vi "Set Magnet.vi"(4 "Mode":T2, 6 "Axis":T1, 8 "error in (no error)":errorcluster, 9 "Target Rate (T/min)":dbl, 10 "Target Field (T)":dbl, 11 "instrument.PPMS2 in":refnum<class "instrument.PPMS2.lvclass">) -> (0 "error out":errorcluster, 3 "instrument.PPMS2 out":refnum<class "instrument.PPMS2.lvclass">)   [LabVIEW 2019, in "instrument.PPMS2.lvclass"]
uses:
  instrument.PPMS2.lvclass
  <userlib>/LevyLab/Levylab Instruments/Instrument Types/Cryostat/Typedefs/Magnet Mode--Enum.ctl
  <userlib>/LevyLab/Levylab Instruments/Instrument Types/Cryostat/Typedefs/Magnet Axis--Enum.ctl
  Typedefs/PPMS2.Commands-enum.ctl
  <userlib>/LevyLab/Levylab Instruments/Instrument Types/Cryostat/Typedefs/Set Magnet--cluster.ctl
  d11e231a-c1e5-403b-8add-65da9e1ac210.vi
  d11e231a-c1e5-403b-8add-65da9e1ac210.vi/1872bd40-8905-4030-a4f5-2c54e5c49330.vi
  <userlib>/LevyLab/Levylab Instruments/SMOs/RemoteControl/API/Remote Client.vi
  <userlib>/LevyLab/Levylab Instruments/Instrument Types/Cryostat/Instrument.Cryostat.lvclass
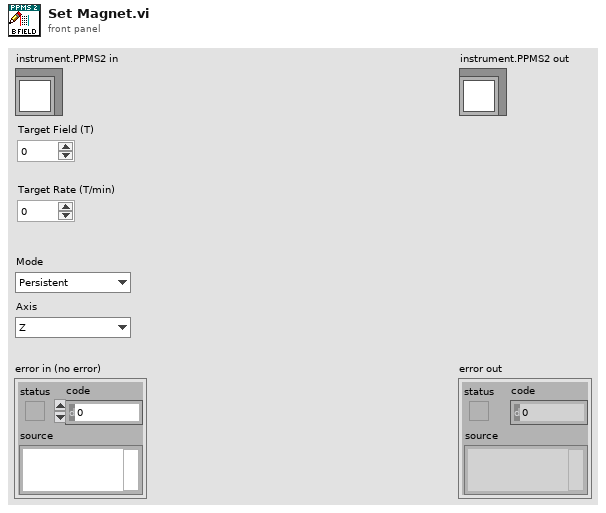
[diagram p1: front panel]
types:
  T1 = typedef "Instrument.Cryostat.lvclass/Magnet Axis--Enum.ctl" = enum16{"Z", "X", "Y"}
  T2 = typedef "Instrument.Cryostat.lvclass/Magnet Mode--Enum.ctl" = enum16{"Persistent", "Driven"}
  T3 = typedef "Instrument.Cryostat.lvclass/Set Magnet--cluster.ctl" = cluster{"Field (T)":dbl, "Rate (T/min)":dbl, "Axis":T1, "Mode":T2}
  T4 = typedef "instrument.PPMS2.lvclass/PPMS2.Commands-enum.ctl" = enum16{"Get Magnet Field", "Get Helium Level", "Get Temperature", "Get Angle", "Set Magnet Field", "Set Temperature", "Set Angle", "getAll"}
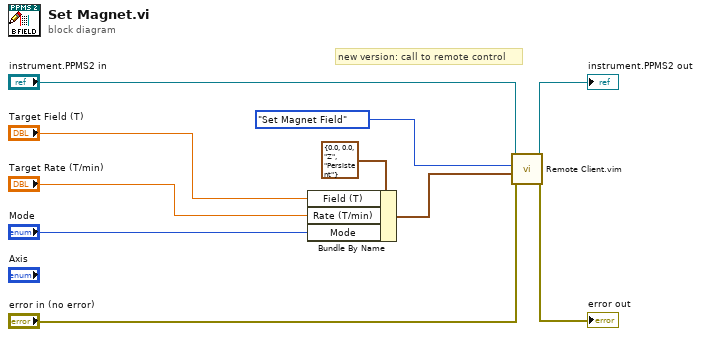
[diagram p0: block diagram]
diagram:
  # "new version: call to remote control"
  n1 = Bundle By Name(cluster=T3 {"Field (T)"=0.0, "Rate (T/min)"=0.0, "Axis"=enum."Z", "Mode"=enum."Persistent"} ("Set Magnet Field"), "Field (T)"="Target Field (T)", "Rate (T/min)"="Target Rate (T/min)", "Mode"="Mode") -> (w5:T3)
  n2 = call "Remote Client.vim"("error in (no error)"="error in (no error)", "Data"=w5, "Command"=PPMS2.Commands-enum."Set Magnet Field" ("Enum"), "Instrument in"="instrument.PPMS2 in") -> ("error out"=→"error out":errorcluster, "Instrument out"=→"instrument.PPMS2 out":refnum<class "instrument.PPMS2.lvclass">)  [unwired: 4 in, 2 out]
